vi "Reset.vi"(8 "error in (no error)":errorcluster, 11 "Agilent DMM in":refnum<class "Agilent DMM.lvclass">) -> (0 "error out":errorcluster, 3 "Agilent DMM out":refnum<class "Agilent DMM.lvclass">)   [LabVIEW 2020, in "Agilent DMM.lvclass"]
uses:
  Agilent DMM.lvclass
  Agilent DMM.lvclass/Agilent DMM.ctl
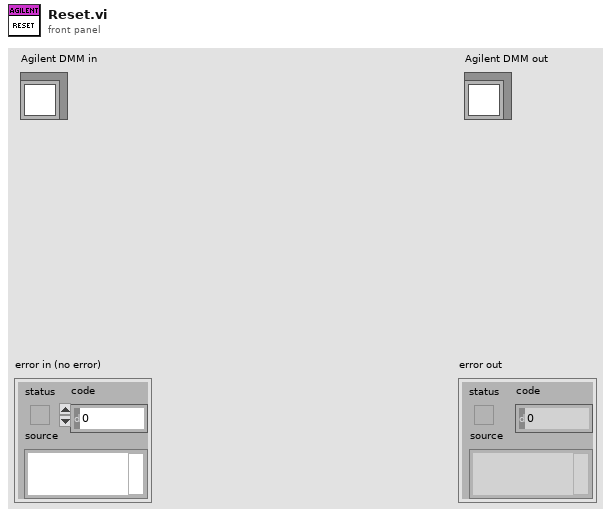
[diagram p1: front panel]
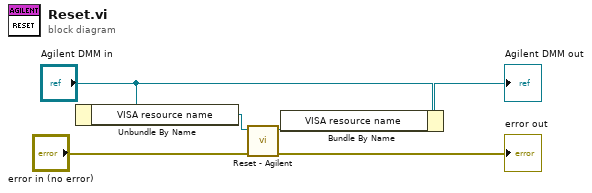
[diagram p0: block diagram]
diagram:
  n1 = Unbundle By Name("Agilent DMM in") -> ("VISA resource name"=w4:refnum<visa-resource-name>)
  n2 = call "Reset - Agilent.vi"("error in (no error)"="error in (no error)", "VISA resource name"=w4) -> ("error out"=→"error out":errorcluster, "VISA resource name out"=w3:refnum<visa-resource-name>)  [unwired: 8 in]
  n3 = Bundle By Name(cluster="Agilent DMM in", "VISA resource name"=w3) -> (→"Agilent DMM out":refnum<class "Agilent DMM.lvclass">)
